vi "Collision Detection global.vi"() -> ()   [LabVIEW 2014]
uses:
  <vilib>/Utility/miscctls.llb/LV3DPointTypeDef.ctl
panel:
  in  "Traverse_XYZ look-out radius (model units)":sgl=100.0
  in  "Reset camera":bool=TRUE
  in  "Force reload geometry":bool
  in  "Draw octree leaf-node boxes":bool
  in  "Highlight tested triangles":bool=TRUE
  in  "Collision marker radius (mm)":sgl=25.0
  in  "Up Direction":T1={"X"=0.0, "Y"=0.0, "Z"=1.0}
  in  "Target":T1
  in  "Camera Position":T1={"X"=4000.0, "Y"=0.0, "Z"=1000.0}
  in  "Model name":string="Elysee_Source1"
  in  "Model octree resolution (model units)":sgl=100.0
  in  "Tunnel octree resolution (model units)":sgl=100.0
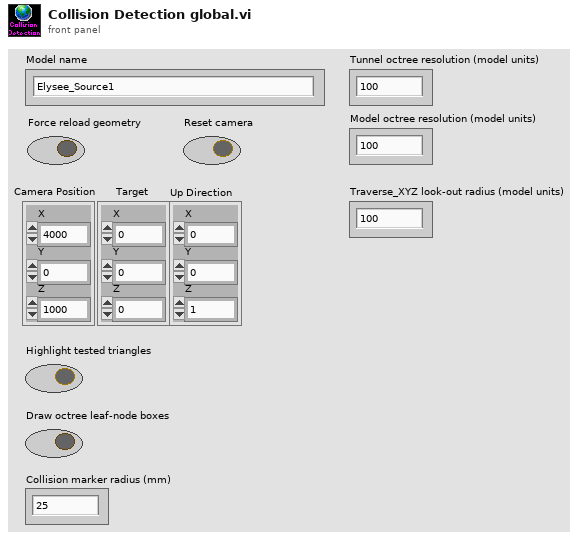
[diagram p1: front panel]
types:
  T1 = typedef "LV3DPointTypeDef.ctl" = cluster{"X":sgl, "Y":sgl, "Z":sgl}
diagram:
